vi "Main Daq routine.vi"() -> ()   [LabVIEW 2025]
uses:
  <vilib>/DAQmx/read.llb/DAQmx Read (Analog 2D DBL NChan NSamp).vi
  <vilib>/DAQmx/miscellaneous.llb/DAQmx Fill In Error Info.vi
  <vilib>/Utility/file.llb/Write Delimited Spreadsheet (DBL).vi
panel:
  out "appended path":path
  out "Duration":dbl
  out "Timer":dbl
  out "HS Daq State":enum16{"Idle", "Start", "Stop", "Running"}(ring)
  out "TC Daq State":enum16{"Idle", "Start", "Stop", "Running"}(ring)
  in  "Enum 3":enum16{"Idle", "Start", "Stop", "Running"}(ring)
  in  "Enum 2":enum16{"Idle", "Start", "Stop", "Running"}(ring)
  out "V/C Daq State":T1(ring)
  in  "Enum":T1(ring)
  in  "Stop HS Daq":bool
  in  "Start HS Daq":bool
  in  "Stop TC Daq":bool
  in  "Start TC Daq":bool
  in  "Stop V/C Daq":bool
  in  "Start V/C Daq":bool
  out "Temperature - samples/Second":i32=2
  out "HS samples/Second":i32=10000
  out "Temperature x16ch":dbl[][](array[numeric]) format="%0.2f"
  out "V/C samples/Second":i32=1000
  out "HS Voltage x4ch":dbl[][](array[numeric])
  out "Voltage and Current":dbl[][](array[numeric])
  in  "EXIT":bool
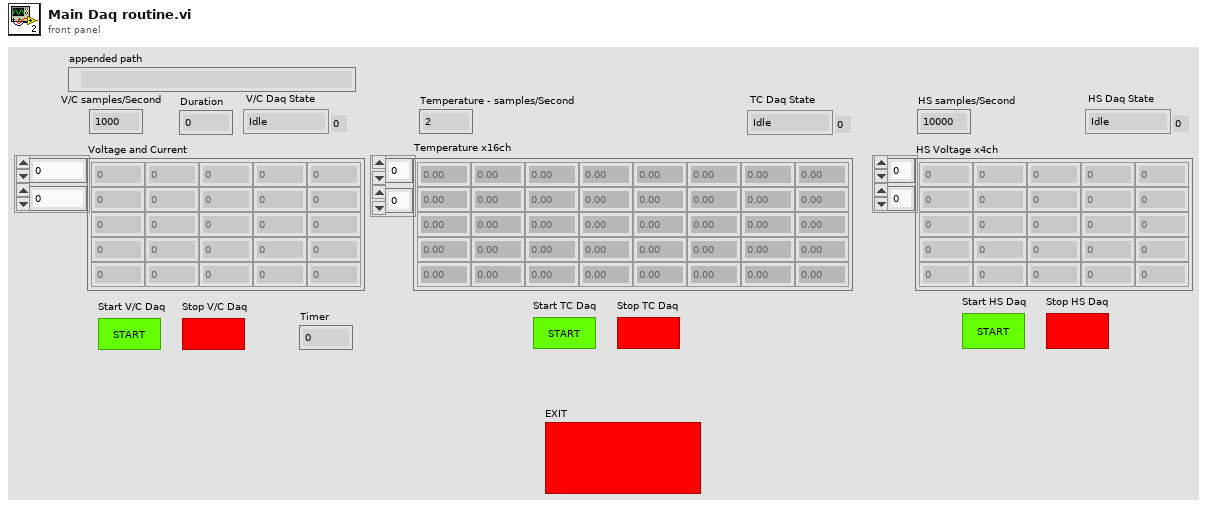
[diagram p1: front panel]
types:
  T1 = enum16{"Idle", "Start", "Stop", "Running", "Record to File"}
  T2 = cluster{"Start HS Daq":bool, "Duration":dbl, "HS Datalog Path":path, "Daq Channels":string, "HS - samples/Second":i32}
  T3 = cluster{"Start TC Daq":bool, "Duration":dbl, "TC Datalog Path":path, "Daq Channels":string, "TC - samples/Second":i32}
  T4 = cluster{"Start TC Daq":bool, "Duration":dbl, "V/C Datalog Path":path, "Daq Channels":string, "V/C - samples/Second":i32}
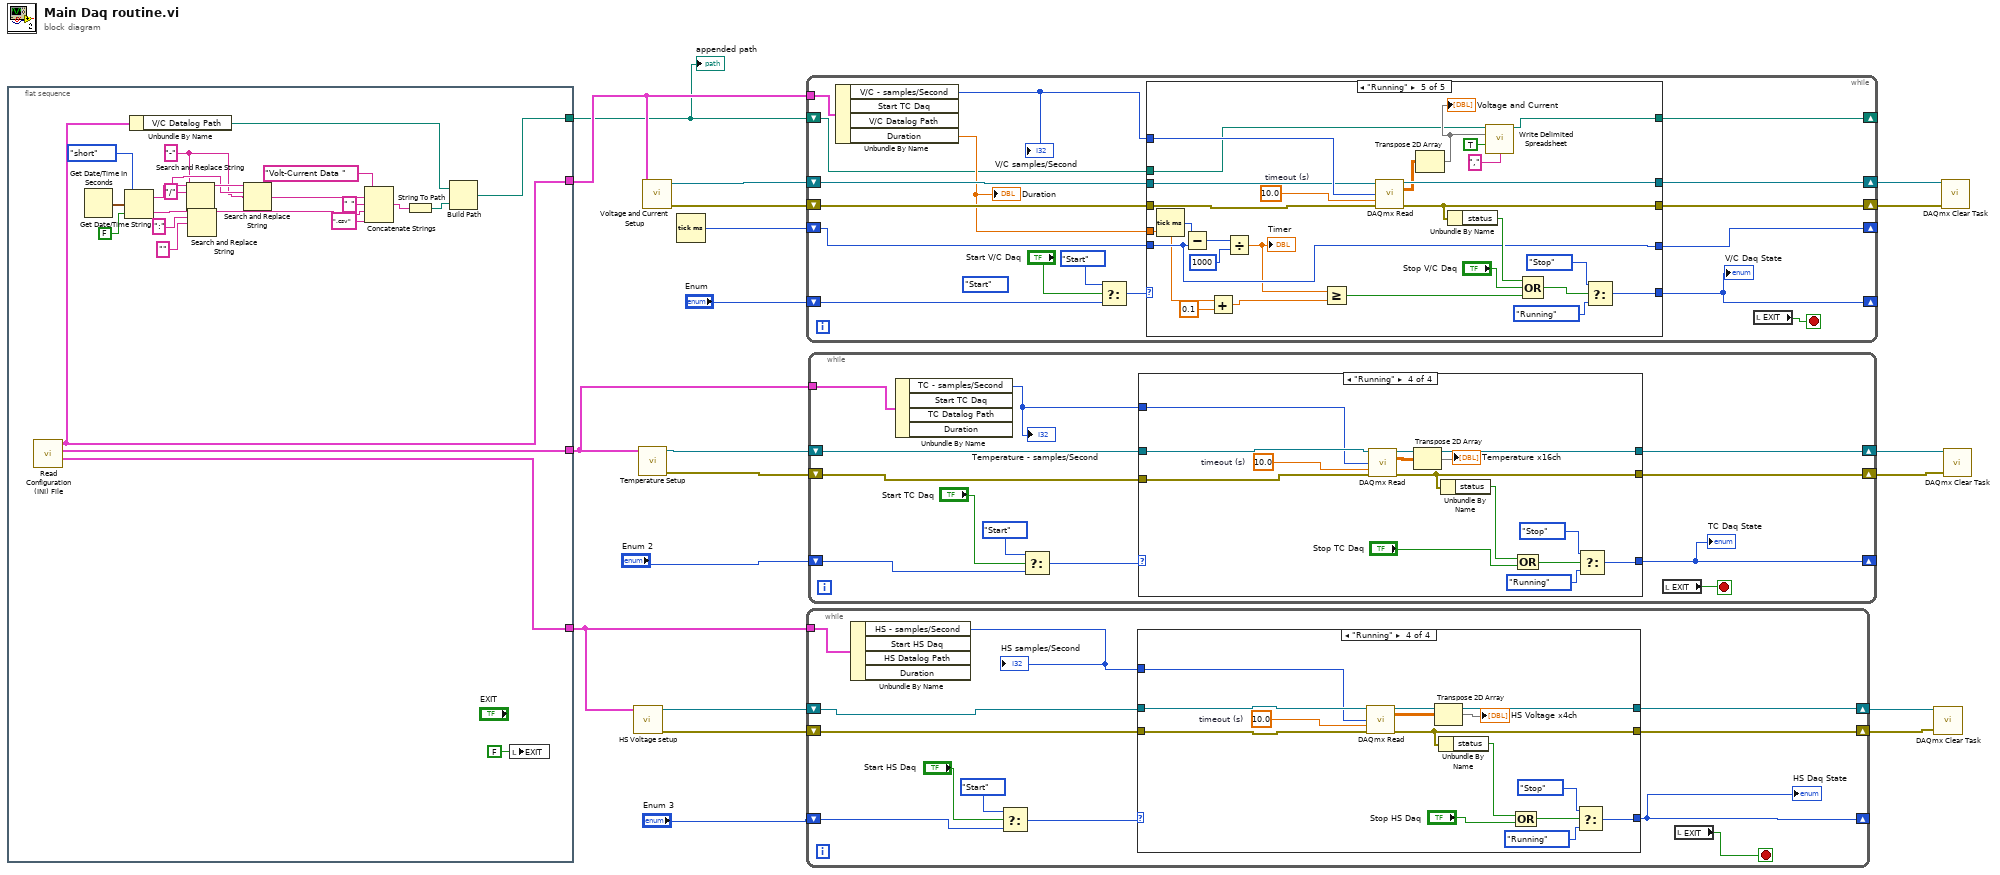
[diagram p0: block diagram]
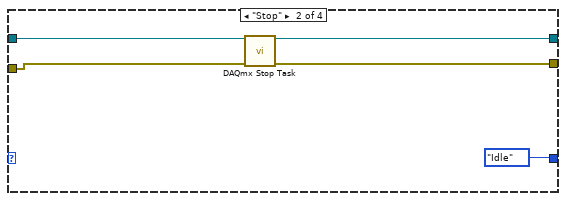
[diagram p3: hidden frame]
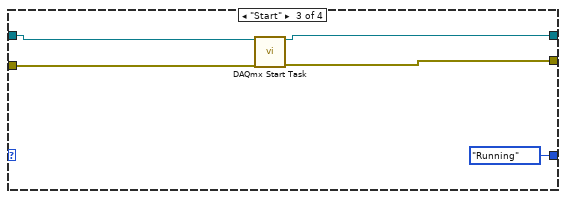
[diagram p4: hidden frame]
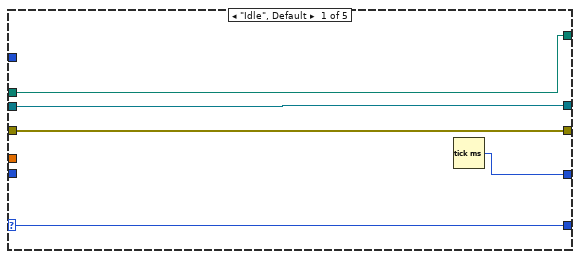
[diagram p5: hidden frame]
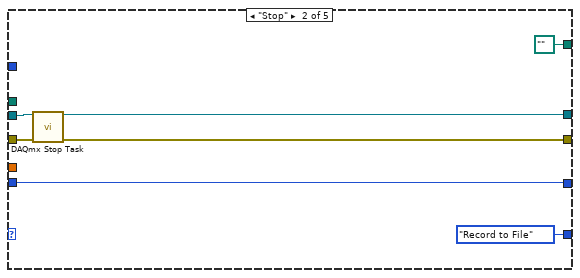
[diagram p6: hidden frame]
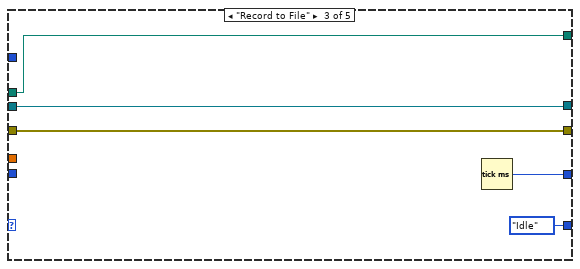
[diagram p7: hidden frame]
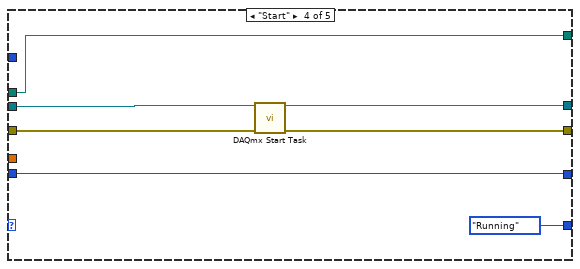
[diagram p8: hidden frame]
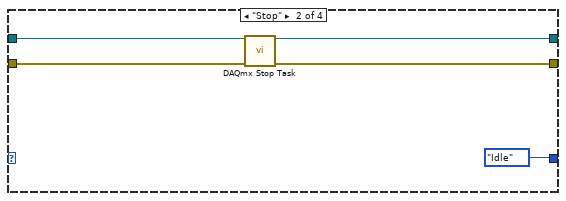
[diagram p10: hidden frame]
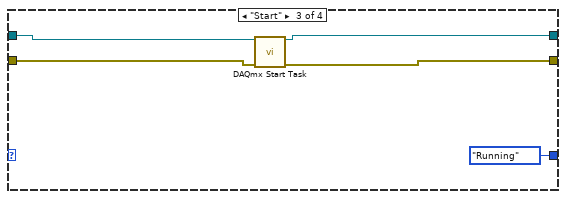
[diagram p11: hidden frame]
diagram:
  n1 = flat-sequence {
    tunnel: [w23] -> w4
    tunnel: [w43] -> w5
    tunnel: [w42] -> w3
    tunnel: [w25] -> w1
    frame #0 {
      w27 = "-" ("replace string (\"\")")
      w28 = "/" ("search string")
      n2 = call "Read Configuration (INI) File.vi"() -> ("HS INI data"=w42:T2, "TC INI data"=w43:T3, "V/C INI data"=w23:T4)  [unwired: 9 in]
      n3 = Get Date/Time In Seconds() -> (seconds since 1Jan1904=w40:timestamp)
      n4 = Get Date/Time String(date format (0)=enum16{"short", "long", "abbreviated"}."short", seconds (now)=w40, want seconds? (F)=FALSE) -> (date string=w31:string, time string=w35:string)
      n5 = Unbundle By Name(w23) -> ("V/C Datalog Path"=w22:path)
      n6 = Search and Replace String(input string=w31, search string=w28, replace string=w27) -> (result string=w29:string)  [unwired: 5 in, 3 out]
      n7 = Search and Replace String(input string=w35, search string=":" ("substring (\"\")"), replace string="" ("replace string (\"\")")) -> (result string=w33:string)  [unwired: 5 in, 3 out]
      n8 = Search and Replace String(input string=w29, search string=w28, replace string=w27) -> (result string=w30:string)  [unwired: 5 in, 3 out]
      n9 = Concatenate Strings("Volt-Current Data " ("string"), w30, " " ("string"), w33, ".csv" ("string")) -> (w21:string)
      n10 = String To Path(string=w21) -> (path=w38:path)
      n11 = Build Path(base path=w22, name or relative path=w38) -> (appended path=w25:path)
      n12 = local write "EXIT"(FALSE ("EXIT")) -> ()
    }
  }
  n13 = call "HS Voltage setup.vi"("HS INI data"=w3) -> ("error out"=w10:errorcluster, "task out"=w9:refnum<k21>)  [unwired: 9 in]
  n14 = call "Temperature Setup.vi"("TC INI data"=w5) -> ("error out"=w12:errorcluster, "task out"=w13:refnum<k21>)  [unwired: 9 in]
  n15 = call "Voltage and Current Setup.vi"("V/C INI data"=w4) -> ("task out"=w20:refnum<k21>, "error out"=w19:errorcluster)  [unwired: 8 in]
  n16 = Tick Count (ms)() -> (millisecond timer value=w2:u32)
  n17 = while {
    tunnel: w4 -> [w52]
    shift-right: [w60] -> w18
    shift-left: w20 -> [w58]
    shift-right: [w59] -> w17
    shift-left: w19 -> [w57]
    shift-right: [w53] -> _
    shift-left: "Enum" -> [w54]
    shift-right: [w47] -> _
    shift-left: w2 -> [w48]
    shift-right: [w44] -> _
    shift-left: w1 -> [w45]
    stop <- w51 stop-if-true
    (unwired) T1."Start" ("Enum")
    n18 = Unbundle By Name(w52) -> ("V/C - samples/Second"=w50:i32, "Duration"=w49:dbl)  [unwired: 2 out]
    "V/C samples/Second" <- w50
    "Duration" <- w49
    n19 = Select(t=T1."Start" ("Enum"), s="Start V/C Daq", f=w54) -> (s? t:f=w56:T1)
    n20 = case shown="\"Running\"" w56 {
      selector: w56 -> [w63 _ _ _ _]
      tunnel: [w65 w72 w77 w82 w111] -> w60
      tunnel: [w64 w71 w76 w81 w110] -> w59
      tunnel: w50 -> [_ _ _ _ w109]
      tunnel: w58 -> [w65 w70 w77 w84 w107]
      tunnel: w57 -> [w64 w69 w76 w83 w108]
      tunnel: [w63 T1."Record to File" ("Enum") T1."Idle" ("Enum") enum16{"Idle", "Start", "Stop", "Running"}."Running" ("Enum") w101] -> w53
      tunnel: w49 -> [_ _ _ _ w93]
      tunnel: w48 -> [_ w68 _ w79 w96]
      tunnel: [w62 w68 w74 w79 w96] -> w47
      tunnel: w45 -> [w61 _ w73 w78 w87]
      tunnel: [w61 path "" ("new file path (Not A Path if cancelled)") w73 w78 w86] -> w44
      frame "Idle", Default {
        n21 = Tick Count (ms)() -> (millisecond timer value=w62:u32)
      }
      frame "Stop" {
        n22 = call <vilib>:"DAQmx Stop Task.vi"("task/channels in"=w70, "error in"=w69) -> ("task out"=w72:refnum<k21>, "error out"=w71:errorcluster)  [unwired: 12 in]
      }
      frame "Record to File" {
        n23 = Tick Count (ms)() -> (millisecond timer value=w74:u32)
      }
      frame "Start" {
        n24 = call <vilib>:"DAQmx Start Task.vi"("task/channels in"=w84, "error in"=w83) -> ("task out"=w82:refnum<k21>, "error out"=w81:errorcluster)  [unwired: 12 in]
      }
      frame "Running" {
        w105 = 10.0  # timeout (s)
        n25 = Tick Count (ms)() -> (millisecond timer value=w98:u32)
        n26 = Subtract(x=w98, y=w96) -> (x-y=w97:u32)
        n27 = Add(x=w93, y=0.1) -> (x+y=w91:dbl)
        n28 = Divide(x=w97, y=u32 1000) -> (x/y=w94:dbl)
        "Timer" <- w94
        n29 = Greater Or Equal?(x=w94, y=w91) -> (x >= y?=w92:bool)
        n30 = call-poly <vilib>:"DAQmx Read.vi"("task/channels in"=w107, "number of samples per channel"=w109, "timeout"=w105, "error in"=w108) -> ("task out"=w111:refnum<k21>, "data"=w104:dbl[][], "error out"=w110:errorcluster)  [unwired: 9 in]
        n31 = Transpose 2D Array(2D array=w104) -> (transposed array=w88:dbl[][])
        "Voltage and Current" <- w88
        n32 = Unbundle By Name(w110) -> ("status"=w106:bool)
        n33 = call-poly <vilib>:"Write Delimited Spreadsheet.vi"("file path (dialog if empty)"=w87, "2D data"=w88, "append to file? (new file:F)"=TRUE, "delimiter (\\t)"="," ("delimiter (\\t)")) -> ("new file path (Not A Path if cancelled)"=w86:path)  [unwired: 10 in, 1 out]
        n34 = Compound Arithmetic op=OR(w106, "Stop V/C Daq", w92) -> (w100:bool)
        n35 = Select(t=enum16{"Idle", "Start", "Stop"}."Stop" ("Enum"), s=w100, f=enum16{"Idle", "Start", "Stop", "Running"}."Running" ("Enum")) -> (s? t:f=w101:enum16{"Idle", "Start", "Stop", "Running"})
      }
    }
    "V/C Daq State" <- w53
    n36 = local read "EXIT"() -> (w51:bool)
  }
  n37 = while {
    tunnel: w3 -> [w114]
    shift-right: [w123] -> w7
    shift-left: w9 -> [w121]
    shift-right: [w122] -> w8
    shift-left: w10 -> [w120]
    shift-right: [w115] -> _
    shift-left: "Enum 3" -> [w116]
    stop <- w113 stop-if-true
    n38 = Unbundle By Name(w114) -> ("HS - samples/Second"=w112:i32)  [unwired: 3 out]
    "HS samples/Second" <- w112
    n39 = Select(t=enum16{"Idle", "Start", "Stop"}."Start" ("Enum"), s="Start HS Daq", f=w116) -> (s? t:f=w118:enum16{"Idle", "Start", "Stop", "Running"})
    n40 = case shown="\"Running\"" w118 {
      selector: w118 -> [w126 _ _ _]
      tunnel: [w125 w131 w136 w150] -> w123
      tunnel: [w124 w130 w135 w149] -> w122
      tunnel: [w126 enum16{"Idle", "Start", "Stop"}."Idle" ("Enum") enum16{"Idle", "Start", "Stop", "Running"}."Running" ("Enum") w145] -> w115
      tunnel: w121 -> [w125 w128 w133 w141]
      tunnel: w120 -> [w124 w127 w132 w140]
      tunnel: w112 -> [_ _ _ w138]
      frame "Idle", Default {
      }
      frame "Stop" {
        n41 = call <vilib>:"DAQmx Stop Task.vi"("task/channels in"=w128, "error in"=w127) -> ("task out"=w131:refnum<k21>, "error out"=w130:errorcluster)  [unwired: 12 in]
      }
      frame "Start" {
        n42 = call <vilib>:"DAQmx Start Task.vi"("task/channels in"=w133, "error in"=w132) -> ("task out"=w136:refnum<k21>, "error out"=w135:errorcluster)  [unwired: 12 in]
      }
      frame "Running" {
        w147 = 10.0  # timeout (s)
        n43 = call-poly <vilib>:"DAQmx Read.vi"("task/channels in"=w141, "number of samples per channel"=w138, "timeout"=w147, "error in"=w140) -> ("task out"=w150:refnum<k21>, "data"=w142:dbl[][], "error out"=w149:errorcluster)  [unwired: 9 in]
        n44 = Transpose 2D Array(2D array=w142) -> (transposed array=→"HS Voltage x4ch":dbl[][])
        n45 = Unbundle By Name(w149) -> ("status"=w148:bool)
        n46 = Compound Arithmetic op=OR(w148, "Stop HS Daq") -> (w144:bool)
        n47 = Select(t=enum16{"Idle", "Start", "Stop"}."Stop" ("Enum"), s=w144, f=enum16{"Idle", "Start", "Stop", "Running"}."Running" ("Enum")) -> (s? t:f=w145:enum16{"Idle", "Start", "Stop", "Running"})
      }
    }
    "HS Daq State" <- w115
    n48 = local read "EXIT"() -> (w113:bool)
  }
  n49 = while {
    tunnel: w5 -> [w153]
    shift-right: [w161] -> w14
    shift-left: w12 -> [w160]
    shift-right: [w162] -> w15
    shift-left: w13 -> [w159]
    shift-right: [w154] -> _
    shift-left: "Enum 2" -> [w156]
    stop <- w151 stop-if-true
    n50 = Unbundle By Name(w153) -> ("TC - samples/Second"=w152:i32)  [unwired: 3 out]
    "Temperature - samples/Second" <- w152
    n51 = Select(t=enum16{"Idle", "Start", "Stop"}."Start" ("Enum"), s="Start TC Daq", f=w156) -> (s? t:f=w157:enum16{"Idle", "Start", "Stop", "Running"})
    n52 = case shown="\"Running\"" w157 {
      selector: w157 -> [w165 _ _ _]
      tunnel: [w164 w170 w175 w189] -> w162
      tunnel: [w163 w169 w174 w188] -> w161
      tunnel: [w165 enum16{"Idle", "Start", "Stop"}."Idle" ("Enum") enum16{"Idle", "Start", "Stop", "Running"}."Running" ("Enum") w184] -> w154
      tunnel: w159 -> [w164 w167 w172 w178]
      tunnel: w160 -> [w163 w166 w171 w177]
      tunnel: w152 -> [_ _ _ w176]
      frame "Idle", Default {
      }
      frame "Stop" {
        n53 = call <vilib>:"DAQmx Stop Task.vi"("task/channels in"=w167, "error in"=w166) -> ("task out"=w170:refnum<k21>, "error out"=w169:errorcluster)  [unwired: 12 in]
      }
      frame "Start" {
        n54 = call <vilib>:"DAQmx Start Task.vi"("task/channels in"=w172, "error in"=w171) -> ("task out"=w175:refnum<k21>, "error out"=w174:errorcluster)  [unwired: 12 in]
      }
      frame "Running" {
        w186 = 10.0  # timeout (s)
        n55 = call-poly <vilib>:"DAQmx Read.vi"("task/channels in"=w178, "number of samples per channel"=w176, "timeout"=w186, "error in"=w177) -> ("task out"=w189:refnum<k21>, "data"=w181:dbl[][], "error out"=w188:errorcluster)  [unwired: 9 in]
        n56 = Transpose 2D Array(2D array=w181) -> (transposed array=→"Temperature x16ch":dbl[][])
        n57 = Unbundle By Name(w188) -> ("status"=w187:bool)
        n58 = Compound Arithmetic op=OR(w187, "Stop TC Daq") -> (w183:bool)
        n59 = Select(t=enum16{"Idle", "Start", "Stop"}."Stop" ("Enum"), s=w183, f=enum16{"Idle", "Start", "Stop", "Running"}."Running" ("Enum")) -> (s? t:f=w184:enum16{"Idle", "Start", "Stop", "Running"})
      }
    }
    "TC Daq State" <- w154
    n60 = local read "EXIT"() -> (w151:bool)
  }
  n61 = call <vilib>:"DAQmx Clear Task.vi"("task in"=w7, "error in"=w8) -> ()  [unwired: 13 in, 1 out]
  n62 = call <vilib>:"DAQmx Clear Task.vi"("task in"=w18, "error in"=w17) -> ()  [unwired: 13 in, 1 out]
  n63 = call <vilib>:"DAQmx Clear Task.vi"("task in"=w15, "error in"=w14) -> ()  [unwired: 13 in, 1 out]
  "appended path" <- w1
